vi "Read.vi"(8 "error in (no error)":errorcluster, 9 "delta connection? (F)":bool, 11 "number of modules":i16) -> (0 "error out":errorcluster, 2 "Data Array":sgl[](array[numeric]) format="%.2f")   [LabVIEW 2017, in "MCSA_9065_API.lvlib"]
uses:
  <vilib>/addons/InsightCM/Devices/Shared/Mcsa/Fpga/McsaAcquire/subVIs/McsaAPI_9065/MCSA_9065_API.lvlib
  <vilib>/eio/EIONode/EIONode.xnode
  <vilib>/rvi/eio/common/nirviEmuTemplateMethod_errors.vi
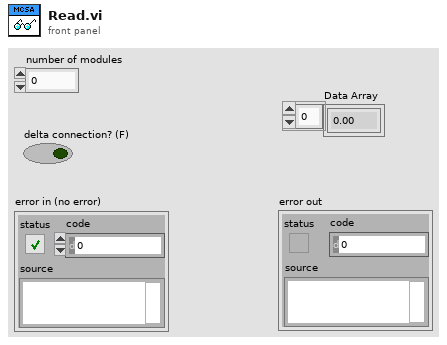
[diagram p1: front panel]
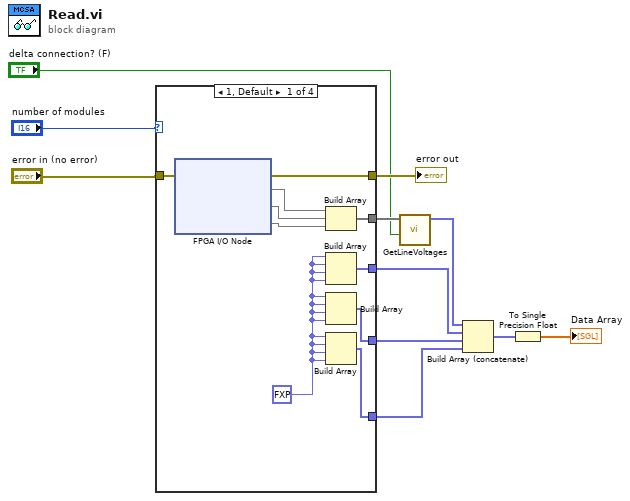
[diagram p0: block diagram]
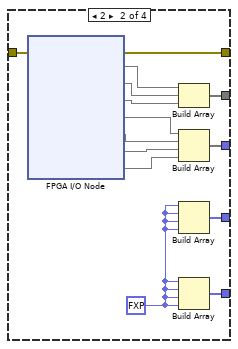
[diagram p2: hidden frame]
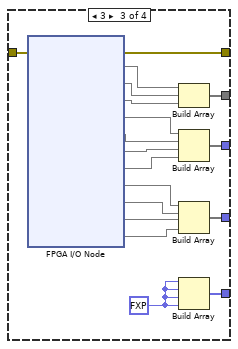
[diagram p3: hidden frame]
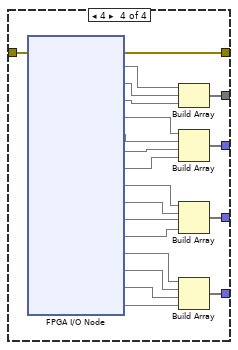
[diagram p4: hidden frame]
diagram:
  n1 = case shown="1, Default" "number of modules" {
    tunnel: "error in (no error)" -> [w18 w32 w50 w71]
    tunnel: [w17 w31 w49 w70] -> w11
    tunnel: [w16 w30 w48 w69] -> w10
    tunnel: [w15 w22 w40 w62] -> w9
    tunnel: [w14 w29 w47 w68] -> w8
    tunnel: [w13 w28 w46 w67] -> w7
    frame 1, Default {
      w12 = fxp<+/-,24,7> 0.0 ("Mod1/AI2")
      n2 = xnode "FPGA I/O Node"("error in"=w18) -> ("error out"=w17:errorcluster, "Mod1/AI0"=w19, "Mod1/AI1"=w21, "Mod1/AI2"=w20)  [unwired: 3 in, 3 out]
      n3 = Build Array(w19, w21, w20) -> (w16:void[])
      n4 = Build Array(w12, w12, w12, w12) -> (w15:fxp<+/-,24,7>[])
      n5 = Build Array(w12, w12, w12, w12) -> (w14:fxp<+/-,24,7>[])
      n6 = Build Array(w12, w12, w12, w12) -> (w13:fxp<+/-,24,7>[])
    }
    frame 2 {
      w27 = fxp<+/-,24,7> 0.0 ("Mod1/AI2")
      n7 = xnode "FPGA I/O Node"("error in"=w32) -> ("error out"=w31:errorcluster, "Mod1/AI0"=w33, "Mod1/AI1"=w35, "Mod1/AI2"=w34, "Mod2/AI0"=w26, "Mod2/AI1"=w25, "Mod2/AI2"=w24, "Mod2/AI3"=w23)  [unwired: 7 in, 7 out]
      n8 = Build Array(w33, w35, w34) -> (w30:void[])
      n9 = Build Array(w26, w25, w24, w23) -> (w22:void[])
      n10 = Build Array(w27, w27, w27, w27) -> (w29:fxp<+/-,24,7>[])
      n11 = Build Array(w27, w27, w27, w27) -> (w28:fxp<+/-,24,7>[])
    }
    frame 3 {
      w45 = fxp<+/-,24,7> 0.0 ("Mod1/AI2")
      n12 = xnode "FPGA I/O Node"("error in"=w50) -> ("error out"=w49:errorcluster, "Mod1/AI0"=w51, "Mod1/AI1"=w53, "Mod1/AI2"=w52, "Mod2/AI0"=w44, "Mod2/AI1"=w43, "Mod2/AI2"=w42, "Mod2/AI3"=w41, "Mod3/AI0"=w39, "Mod3/AI1"=w38, "Mod3/AI2"=w37, "Mod3/AI3"=w36)  [unwired: 11 in, 11 out]
      n13 = Build Array(w51, w53, w52) -> (w48:void[])
      n14 = Build Array(w44, w43, w42, w41) -> (w40:void[])
      n15 = Build Array(w39, w38, w37, w36) -> (w47:void[])
      n16 = Build Array(w45, w45, w45, w45) -> (w46:fxp<+/-,24,7>[])
    }
    frame 4 {
      n17 = xnode "FPGA I/O Node"("error in"=w71) -> ("error out"=w70:errorcluster, "Mod1/AI0"=w72, "Mod1/AI1"=w74, "Mod1/AI2"=w73, "Mod2/AI0"=w66, "Mod2/AI1"=w65, "Mod2/AI2"=w64, "Mod2/AI3"=w63, "Mod3/AI0"=w61, "Mod3/AI1"=w60, "Mod3/AI2"=w59, "Mod3/AI3"=w58, "Mod4/AI0"=w57, "Mod4/AI1"=w56, "Mod4/AI2"=w55, "Mod4/AI3"=w54)  [unwired: 15 in, 15 out]
      n18 = Build Array(w72, w74, w73) -> (w69:void[])
      n19 = Build Array(w66, w65, w64, w63) -> (w62:void[])
      n20 = Build Array(w61, w60, w59, w58) -> (w68:void[])
      n21 = Build Array(w57, w56, w55, w54) -> (w67:void[])
    }
  }
  "error out" <- w11
  n22 = call <vilib>:"GetLineVoltages.vi"("delta connection? (F)"="delta connection? (F)", "original voltages"=w10) -> ("line or phase voltages"=w2:fxp<+/-,25,11>[])  [unwired: 9 in]
  n23 = Build Array (concatenate)(w2, w9, w8, w7) -> (w6:fxp<+/-,28,11>[])
  n24 = To Single Precision Float(number=w6) -> (single precision float=→"Data Array":sgl[])
